vi "Write Sequence Steps.vi"(10 "Steps":refnum<class "IModel.lvclass">[](array[class]), 11 "SequencingModel in":refnum<class "SequencingModel.lvclass">) -> (3 "SequencingModel out":refnum<class "SequencingModel.lvclass">)   [LabVIEW 2017, in "SequencingModel.lvlib" / "SequencingModel.lvclass"]
uses:
  <vilib>/gpm_packages/@cs/example/Dynamic Viewables/SequencingModel/SequencingModel.lvclass
  <vilib>/gpm_packages/@cs/mva-core/Source/IModel/IModel/IModel.lvclass
  <vilib>/gpm_packages/@cs/example/Dynamic Viewables/SequencingModel/SequencingModel.lvclass/SequencingModel.ctl
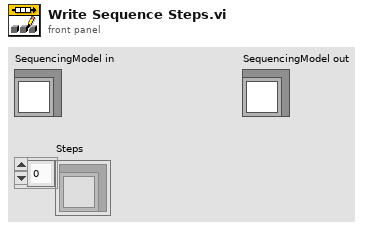
[diagram p1: front panel]
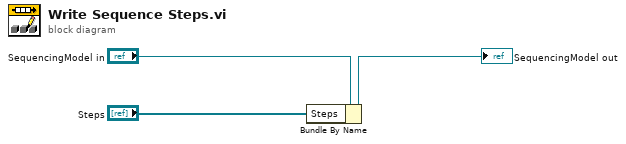
[diagram p0: block diagram]
diagram:
  n1 = Bundle By Name(cluster="SequencingModel in", "Steps"="Steps") -> (→"SequencingModel out":refnum<class "SequencingModel.lvclass">)
